vi "StandAloneTransient_NIDCPOWER_PSU_POWER_CYCLE_V1.vi"(7 "NIDCPOWER_VOLT_CONF":dbl, 8 "error in (no error)":errorcluster, 9 "milliseconds to wait":u32, 10 "NIDCPOWER_CHAN_CONF":string, 11 "IVI Refnum in":refnum<k15>) -> (0 "error out":errorcluster)   [LabVIEW 2019]
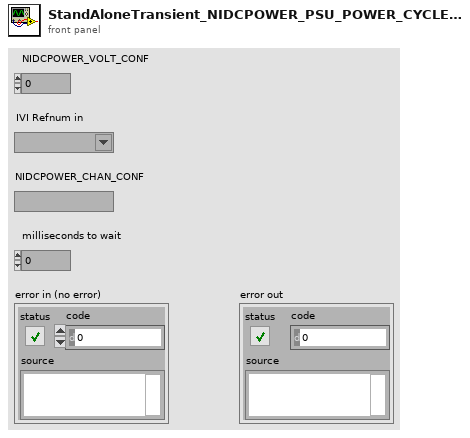
[diagram p1: front panel]
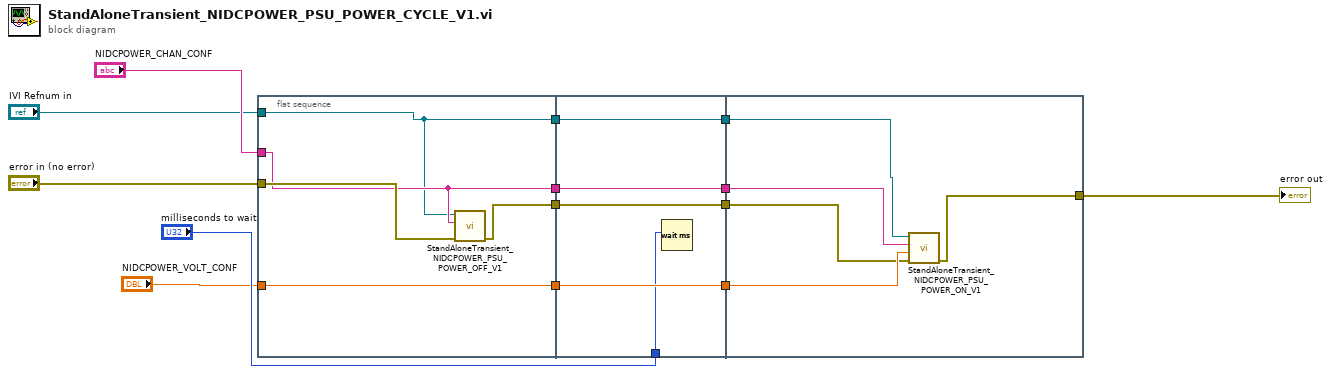
[diagram p0: block diagram]
diagram:
  n1 = flat-sequence {
    tunnel: "IVI Refnum in" -> [w16]
    tunnel: "error in (no error)" -> [w18]
    tunnel: [w15] -> w14
    tunnel: [w17] -> w13
    tunnel: [w16] -> w12
    tunnel: "NIDCPOWER_CHAN_CONF" -> [w17]
    tunnel: [w19] -> w11
    tunnel: "NIDCPOWER_VOLT_CONF" -> [w19]
    tunnel: [w24] -> w10
    tunnel: w14 -> [w24]
    tunnel: [w23] -> w9
    tunnel: w13 -> [w23]
    tunnel: w12 -> [w22]
    tunnel: [w22] -> w8
    tunnel: [w21] -> w7
    tunnel: w11 -> [w21]
    tunnel: "milliseconds to wait" -> [w20]
    tunnel: w10 -> [w26]
    tunnel: w9 -> [w28]
    tunnel: w8 -> [w27]
    tunnel: [w25] -> w3
    tunnel: w7 -> [w29]
    frame #0 {
      n2 = call "StandAloneTransient_NIDCPOWER_PSU_POWER_OFF_V1.vi"("error in"=w18, "channel name"=w17, "resource name"=w16) -> ("eRROR OUT"=w15:errorcluster)  [unwired: 8 in]
    }
    frame #1 {
      n3 = Wait (ms)(milliseconds to wait=w20) -> ()  [unwired: 1 out]
    }
    frame #2 {
      n4 = call "StandAloneTransient_NIDCPOWER_PSU_POWER_ON_V1.vi"("error in"=w26, "voltage level"=w29, "channel name"=w28, "resource name"=w27) -> ("error out"=w25:errorcluster)  [unwired: 6 in, 1 out]
    }
  }
  "error out" <- w3
